vi "DHE_DescribeDriverErrors.vi"(0 "message":string, 2 "OK message":string="DONE", 3 "error in (no error)":errorcluster) -> (7 "error?":bool, 8 "astroerrors":string, 10 "error out":errorcluster)   [LabVIEW 2016]
doc: "This subVI tests the error status output of one or more low-level functions or subVIs that output a numeric error code, and creates an error out cluster that can be wired to the Simple or General Error Handler in order to identify the error and describe it to the user.\n\nThe error in cluster is tested first. If error? is no-error, the elements of the error codes array are tested next for non-zero values. The first error found terminates the test, and error out identifies that error. Use a Build Array function to assemble the individual error codes.\n\nYou can optionally use the source messages string to pass on the source of the error. Enter one line of text for each element of the error codes array. \n\nThe error? status is TRUE on any error."
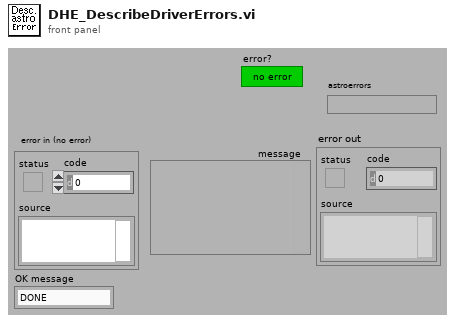
[diagram p1: front panel]
types:
  T1 = typedef "DatabaseHand_RefNum.ctl" = refnum<vi>
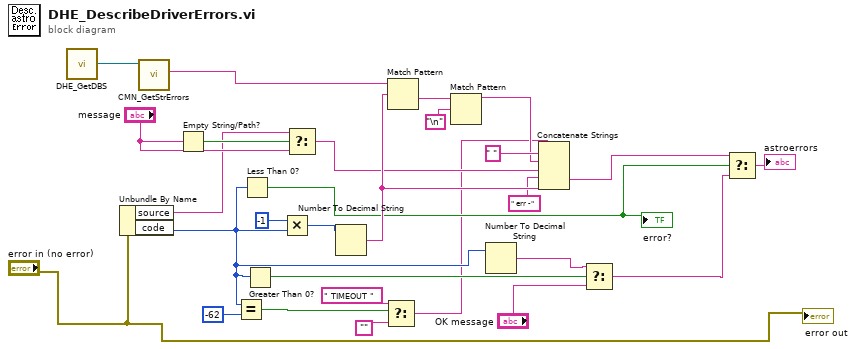
[diagram p0: block diagram]
diagram:
  n1 = call "DHE_GetDBS.vi"() -> ("DHE_DBSRef"=w2:T1)  [unwired: 9 out]
  n2 = Unbundle By Name("error in (no error)") -> ("source"=w17:string, "code"=w13:i32)
  n3 = call "CMN_GetStrErrors.vi"("Database RefNum"=w2) -> ("errors"=w3:string)  [unwired: 10 out]
  n4 = Empty String/Path?(string/path="message") -> (empty?=w19:bool)
  n5 = Equal?(x=w13, y=-62) -> (x = y?=w11:bool)
  n6 = Less Than 0?(x=w13) -> (x < 0?=w21:bool)
  "error?" <- w21
  n7 = Greater Than 0?(x=w13) -> (x > 0?=w14:bool)
  n8 = Multiply(x=-1, y=w13) -> (x*y=w4:i32)
  n9 = Select(t=w17, s=w19, f="message") -> (s? t:f=w16:string)
  n10 = Number To Decimal String(number=w4) -> (decimal integer string=w24:string)  [unwired: 1 out]
  n11 = Select(t=" TIMEOUT ", s=w11, f="") -> (s? t:f=w8:string)
  n12 = Match Pattern(string=w3, regular expression=w24) -> (after substring=w26:string)  [unwired: 4 out]
  n13 = Match Pattern(string=w26, regular expression="\n") -> (before substring=w15:string)  [unwired: 4 out]
  n14 = Number To Decimal String(number=w13) -> (decimal integer string=w5:string)  [unwired: 1 out]
  n15 = Concatenate Strings(w8, " ", w15, w16, " err -", w24) -> (w28:string)
  n16 = Select(t=w5, s=w14, f="OK message") -> (s? t:f=w7:string)
  n17 = Select(t=w28, s=w21, f=w7) -> (s? t:f=→"astroerrors":string)
  "error out" <- "error in (no error)"
